vi "CheckDataOutFullLayer.vi"(0 "InputEventWord":u32[](array[numeric]), 7 "ID list":u32[](array[numeric])=[47735, 47735, 49079, 47223, 48247] format="%x") -> (4 "DataChip1 OK?":bool, 6 "DataChip2 OK?":bool, 8 "DataChip3 OK?":bool, 10 "DataChip4 OK?":bool)   [LabVIEW 2015, in "VIPM2.lvlib"]
uses:
  VIPM2.lvlib
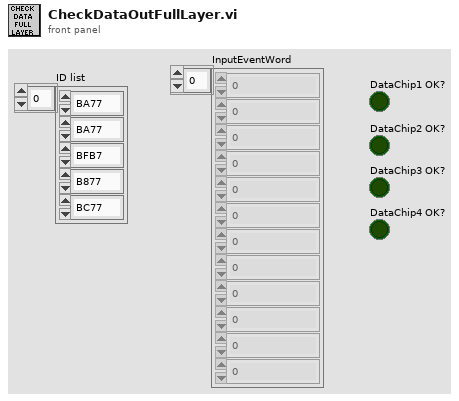
[diagram p1: front panel]
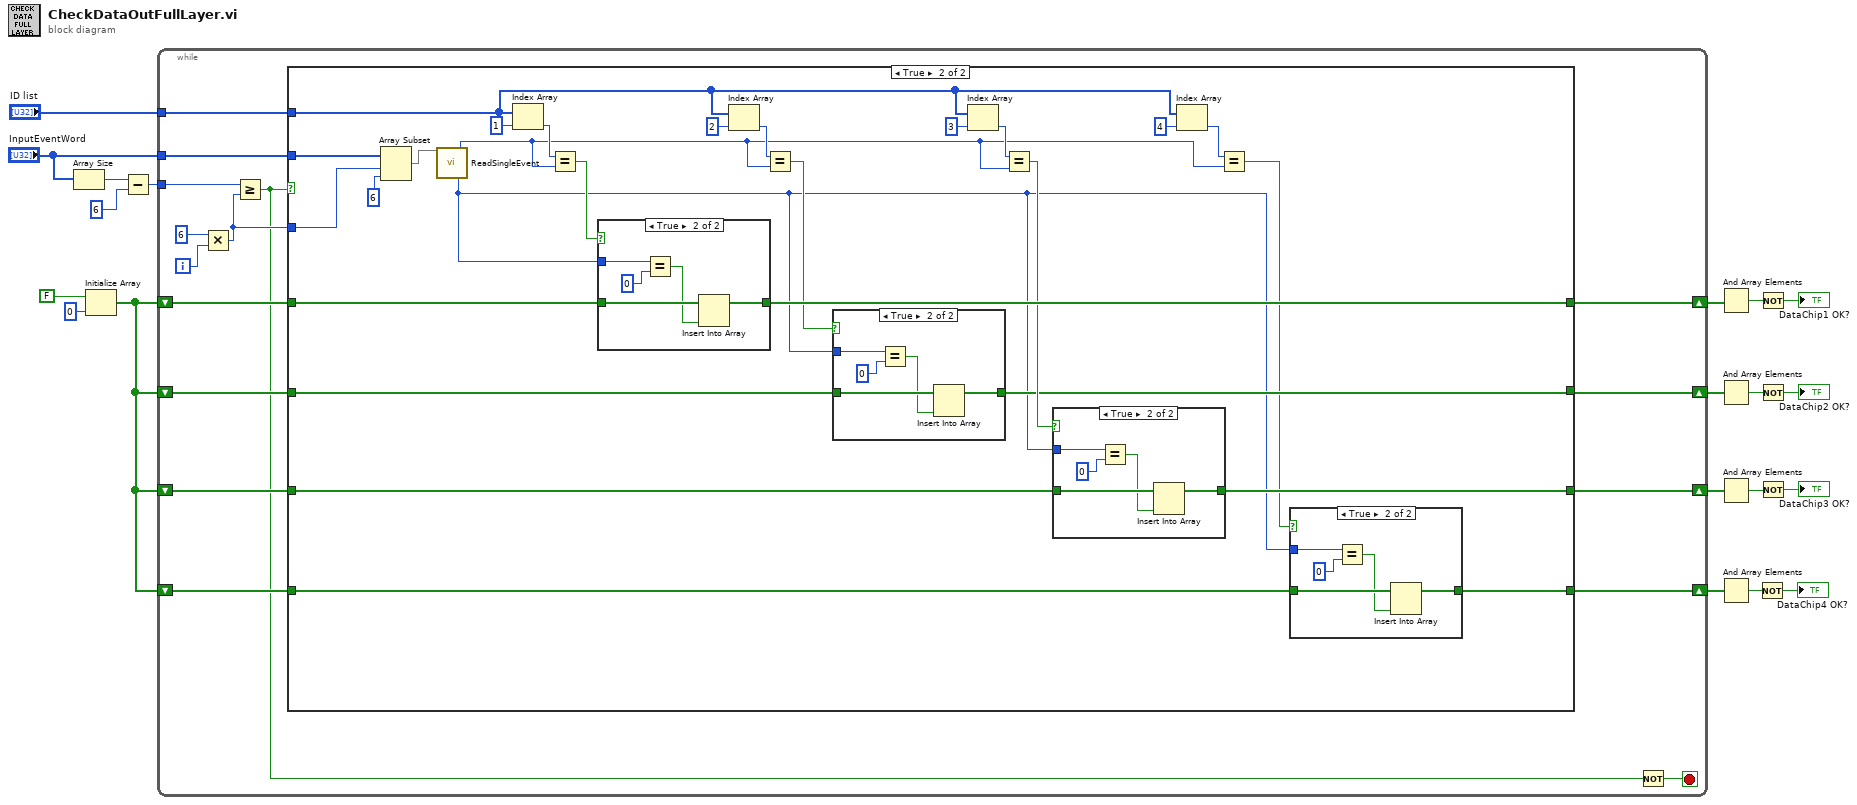
[diagram p0: block diagram]
diagram:
  n1 = Array Size(array="InputEventWord") -> (size(s)=w19:i32)
  n2 = Initialize Array(FALSE, 0 ("dimension size")) -> (w13:bool[])
  n3 = Subtract(x=w19, y=6) -> (x-y=w17:i32)
  n4 = while {
    tunnel: "InputEventWord" -> [w36]
    tunnel: w17 -> [w33]
    tunnel: "ID list" -> [w31]
    shift-right: [w29] -> w12
    shift-left: w13 -> [w30]
    shift-right: [w27] -> w11
    shift-left: w13 -> [w28]
    shift-right: [w25] -> w10
    shift-left: w13 -> [w26]
    shift-right: [w23] -> w9
    shift-left: w13 -> [w24]
    i -> [w34]
    stop <- w21 stop-if-true
    n5 = Multiply(x=6 ("length"), y=w34) -> (x*y=w32:i32)
    n6 = Greater Or Equal?(x=w33, y=w32) -> (x >= y?=w22:bool)
    n7 = case shown="True" w22 {
      tunnel: w36 -> [_ w67]
      tunnel: w32 -> [_ w65]
      tunnel: w31 -> [_ w63]
      tunnel: w30 -> [w40 w52]
      tunnel: [w40 w51] -> w29
      tunnel: w28 -> [w39 w50]
      tunnel: [w39 w47] -> w27
      tunnel: w26 -> [w38 w46]
      tunnel: [w38 w45] -> w25
      tunnel: w24 -> [w37 w42]
      tunnel: [w37 w41] -> w23
      frame False {
      }
      frame True {
        n8 = Array Subset(array=w67, index=w65, length=6) -> (w64:u32[])
        n9 = call "ReadSingleEvent.vi"("InputEventWord"=w64) -> ("ChipID"=w54:u16, "ADCTrigPix"=w43:u32)  [unwired: 8 in, 5 out]
        n10 = Index Array(array=w63, index=1) -> (element=w58:u32)
        n11 = Equal?(x=w58, y=w54) -> (x = y?=w53:bool)
        n12 = case shown="True" w53 {
          tunnel: w52 -> [w86 w91]
          tunnel: w43 -> [_ w89]
          tunnel: [w86 w87] -> w51
          frame False {
          }
          frame True {
            n13 = Equal?(x=w89, y=u32 0) -> (x = y?=w88:bool)
            n14 = Insert Into Array(array=w91, new element=w88) -> (w87:bool[])  [unwired: 1 in]
          }
        }
        n15 = Index Array(array=w63, index=2) -> (element=w57:u32)
        n16 = Equal?(x=w57, y=w54) -> (x = y?=w49:bool)
        n17 = case shown="True" w49 {
          tunnel: w50 -> [w80 w85]
          tunnel: w43 -> [_ w83]
          tunnel: [w80 w81] -> w47
          frame False {
          }
          frame True {
            n18 = Equal?(x=w83, y=u32 0) -> (x = y?=w82:bool)
            n19 = Insert Into Array(array=w85, new element=w82) -> (w81:bool[])  [unwired: 1 in]
          }
        }
        n20 = Index Array(array=w63, index=3) -> (element=w56:u32)
        n21 = Equal?(x=w56, y=w54) -> (x = y?=w48:bool)
        n22 = case shown="True" w48 {
          tunnel: w46 -> [w74 w79]
          tunnel: w43 -> [_ w77]
          tunnel: [w74 w75] -> w45
          frame False {
          }
          frame True {
            n23 = Equal?(x=w77, y=u32 0) -> (x = y?=w76:bool)
            n24 = Insert Into Array(array=w79, new element=w76) -> (w75:bool[])  [unwired: 1 in]
          }
        }
        n25 = Index Array(array=w63, index=4) -> (element=w55:u32)
        n26 = Equal?(x=w55, y=w54) -> (x = y?=w44:bool)
        n27 = case shown="True" w44 {
          tunnel: w42 -> [w68 w73]
          tunnel: w43 -> [_ w71]
          tunnel: [w68 w69] -> w41
          frame False {
          }
          frame True {
            n28 = Equal?(x=w71, y=u32 0) -> (x = y?=w70:bool)
            n29 = Insert Into Array(array=w73, new element=w70) -> (w69:bool[])  [unwired: 1 in]
          }
        }
      }
    }
    n30 = Not(x=w22) -> (.not. x?=w21:bool)
  }
  n31 = And Array Elements(Boolean array=w12) -> (logical AND=w8:bool)
  n32 = And Array Elements(Boolean array=w11) -> (logical AND=w3:bool)
  n33 = And Array Elements(Boolean array=w10) -> (logical AND=w2:bool)
  n34 = And Array Elements(Boolean array=w9) -> (logical AND=w1:bool)
  n35 = Not(x=w1) -> (.not. x?=→"DataChip4 OK?":bool)
  n36 = Not(x=w8) -> (.not. x?=→"DataChip1 OK?":bool)
  n37 = Not(x=w3) -> (.not. x?=→"DataChip2 OK?":bool)
  n38 = Not(x=w2) -> (.not. x?=→"DataChip3 OK?":bool)
